vi "nanocal -- plotstring file manage.vi"(7 "Enum":T1, 8 "all data":cluster{"Array":dbl[], "Array":dbl[]}[](array[cluster]), 10 "header line":string, 11 "full filename":path) -> (1 "plotstring thing":string)   [LabVIEW 2020]
uses:
  nanocal -- plotstring file action.ctl
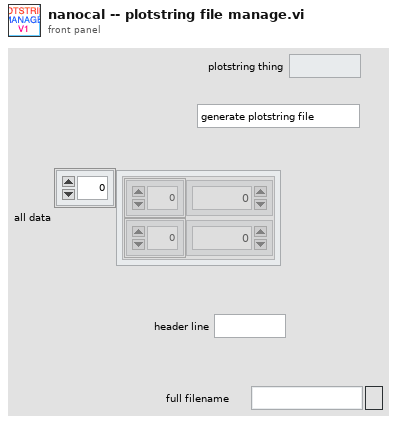
[diagram p1: front panel]
types:
  T1 = typedef "nanocal -- plotstring file action.ctl" = enum16{"generate plotstring file", "generate plotstring thing", ""}
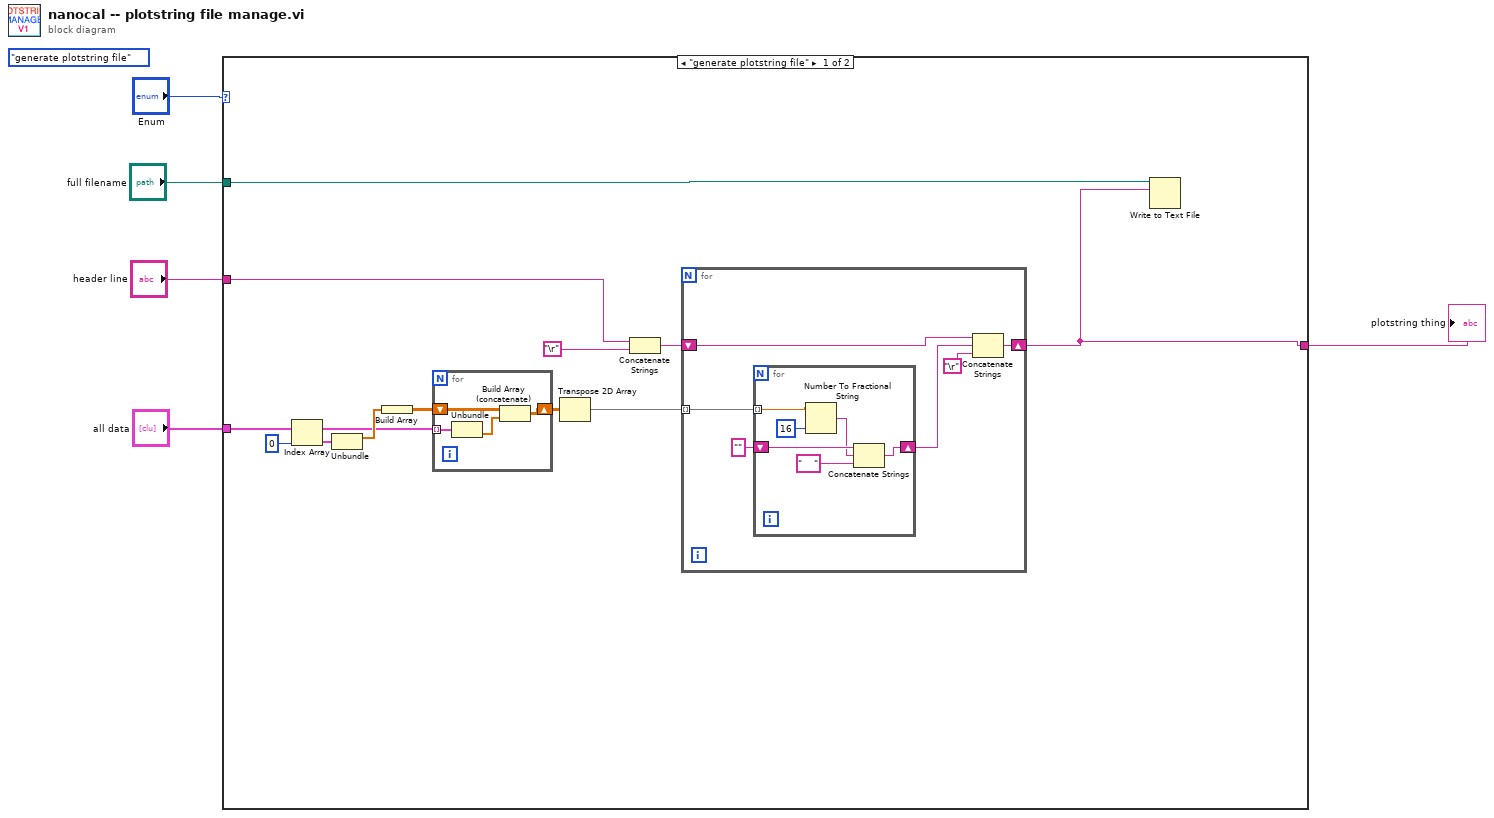
[diagram p0: block diagram]
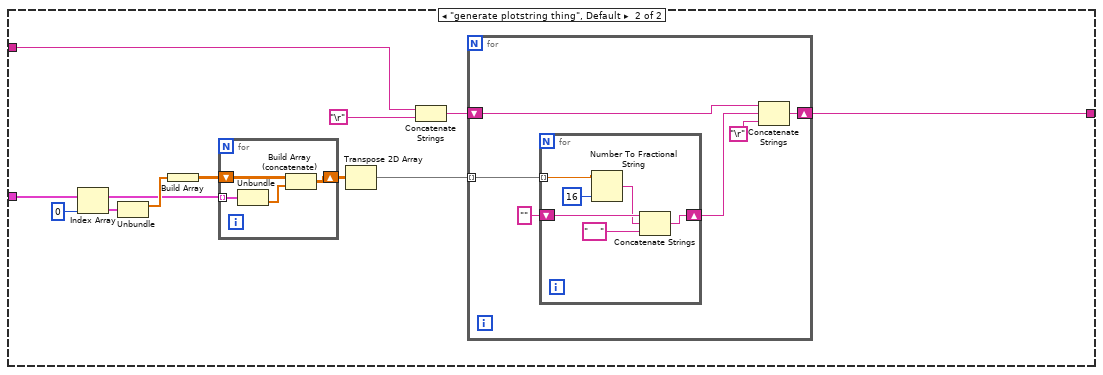
[diagram p2: hidden frame]
diagram:
  (unwired) nanocal_--_plotstring_file_action."generate plotstring file"
  n1 = case shown="\"generate plotstring file\"" "Enum" {
    tunnel: "header line" -> [w9 w36]
    tunnel: "full filename" -> [w8 _]
    tunnel: "all data" -> [w7 w35]
    tunnel: [w6 w34] -> w1
    frame "generate plotstring file" {
      n2 = Index Array(array=w7, index=0) -> (element=w16:cluster{"Array":dbl[], "Array":dbl[]})
      n3 = Unbundle(w16) -> ("Array"=w15:dbl[])  [unwired: 1 out]
      n4 = Build Array(w15) -> (w14:dbl[][])
      n5 = for {
        shift-right: [w31] -> w13
        shift-left: w14 -> [w33]
        tunnel: w7 -> [w30] mode=indexing
        n6 = Unbundle(w30) -> ("Array"=w32:dbl[])  [unwired: 1 out]
        n7 = Build Array (concatenate)(w33, w32) -> (w31:dbl[][])
      }
      n8 = Transpose 2D Array(2D array=w13) -> (transposed array=w12:dbl[][])
      n9 = Concatenate Strings(w9, "\r") -> (w10:string)
      n10 = for {
        shift-right: [w23] -> w6
        shift-left: w10 -> [w22]
        tunnel: w12 -> [w20] mode=indexing
        n11 = for {
          shift-right: [w24] -> w19
          shift-left: "" -> [w29]
          tunnel: w20 -> [w28] mode=indexing
          n12 = Number To Fractional String(number=w28, precision (6)=i16 16) -> (F-format string=w26:string)  [unwired: 2 in]
          n13 = Concatenate Strings(w29, w26, "    ") -> (w24:string)
        }
        n14 = Concatenate Strings(w22, w19, "\r") -> (w23:string)
      }
      n15 = Write to Text File(file (use dialog)=w8, text=w6) -> ()  [unwired: 2 in, 3 out]
    }
    frame "generate plotstring thing", Default {
      n16 = Index Array(array=w35, index=0) -> (element=w43:cluster{"Array":dbl[], "Array":dbl[]})
      n17 = Unbundle(w43) -> ("Array"=w42:dbl[])  [unwired: 1 out]
      n18 = Build Array(w42) -> (w41:dbl[][])
      n19 = for {
        shift-right: [w58] -> w40
        shift-left: w41 -> [w60]
        tunnel: w35 -> [w57] mode=indexing
        n20 = Unbundle(w57) -> ("Array"=w59:dbl[])  [unwired: 1 out]
        n21 = Build Array (concatenate)(w60, w59) -> (w58:dbl[][])
      }
      n22 = Transpose 2D Array(2D array=w40) -> (transposed array=w39:dbl[][])
      n23 = Concatenate Strings(w36, "\r") -> (w37:string)
      n24 = for {
        shift-right: [w50] -> w34
        shift-left: w37 -> [w49]
        tunnel: w39 -> [w47] mode=indexing
        n25 = for {
          shift-right: [w51] -> w46
          shift-left: "" -> [w56]
          tunnel: w47 -> [w55] mode=indexing
          n26 = Number To Fractional String(number=w55, precision (6)=i16 16) -> (F-format string=w53:string)  [unwired: 2 in]
          n27 = Concatenate Strings(w56, w53, "    ") -> (w51:string)
        }
        n28 = Concatenate Strings(w49, w46, "\r") -> (w50:string)
      }
    }
  }
  "plotstring thing" <- w1
